vi "Update Non-SD Channels.vi"(7 "Type":T2, 8 "error in (no error)":errorcluster, 9 "Channel Names":string[](array[string]), 10 "Node Ptr In":T1 format="%.0x", 11 "9402 in":refnum<class "9402.lvclass">) -> (0 "error out":errorcluster, 2 "Node Ptr Out":T1 format="%.0x", 3 "9402 out":refnum<class "9402.lvclass">)   [LabVIEW 2017, in "Modules.lvlib" / "9402.lvclass"]
uses:
  9402.lvclass
  <vilib>/NI Veristand/Custom Device API/Custom Device Channel Type.ctl
  <vilib>/NI Veristand/Custom Device API/Custom Device Item Ref.ctl
  <vilib>/NI Veristand/Custom Device API/Custom Device API.lvlib
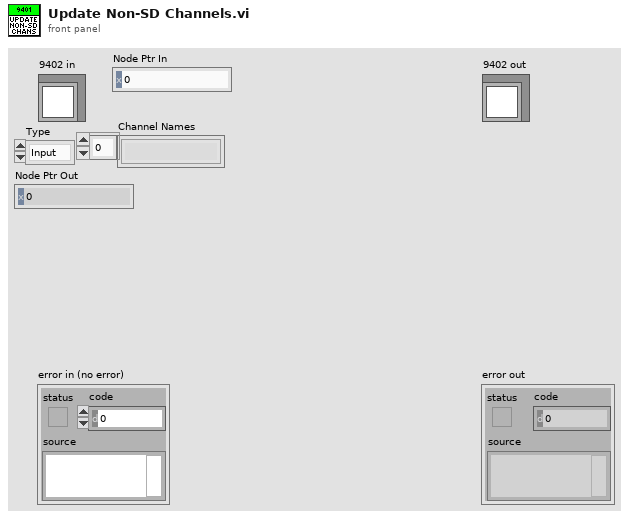
[diagram p1: front panel]
types:
  T1 = typedef "Custom Device API.lvlib/Custom Device Item Ref.ctl" = u64
  T2 = typedef "Custom Device API.lvlib/Custom Device Channel Type.ctl" = enum16{"Input", "Output"}
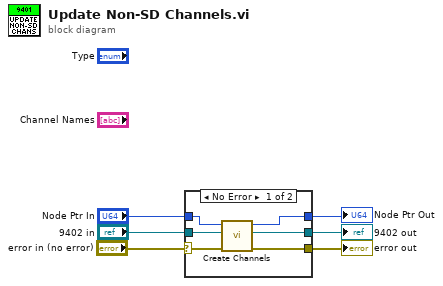
[diagram p0: block diagram]
diagram:
  n1 = case shown="No Error" "error in (no error)" {
    selector: "error in (no error)" -> [w10 w13]
    tunnel: "Node Ptr In" -> [w12 w15]
    tunnel: [w11 w15] -> w5
    tunnel: "9402 in" -> [w9 w14]
    tunnel: [w8 w14] -> w2
    tunnel: [w7 w13] -> w1
    frame No Error {
      n2 = call-dynamic "Create Channels.vi"("error in (no error)"=w10, "RSI Module in"=w9, "Parent Ref in"=w12) -> ("error out"=w7:errorcluster, "RSI Module out"=w8:refnum<class "9402.lvclass">, "Parent Ref out"=w11:T1)  [unwired: 6 in]
    }
    frame Error {
    }
  }
  "error out" <- w1
  "9402 out" <- w2
  "Node Ptr Out" <- w5
